vi "PrepareXYSignals.vi"(8 "error in (no error)":errorcluster, 9 "Parameters":T2={"number of planes"=4, "z step"=1.9999999999999998e-05, "pixel dwell time"=1.0000000000000001e-11, "z frequency"=10.0, "number of pixels"=100, "smooth points"=10, "smooth line"=10, "Sine\nSawtooth"=FALSE, "PointSorting"=0, "Sort Points"=FALSE, "X-pixels"=256.0, "Y-lines"=256.0, "pixelstoµm"=256.0, "zoom"=1.0, "Time offset"=1.0000000000000001e-11} {"zoom" min=0.5 step=0.1; "Y-lines" min=1 step=1; "X-pixels" min=1 step=1; "PointSorting" items=["No Difference", "Every Second Point", "Down / Up"]; "smooth line" min=1; "smooth points" min=1; "number of pixels" min=1; "z frequency" format="%_4g"; "number of planes" min=1}, 10 "DutyCluster":T1 {"Iteration" items=["first iteration", "second iteration"]}, 11 "XYZ Point coordinates (pixels)":dbl[][](array[numeric])) -> (0 "error out":errorcluster, 2 "DutyCluster":T1 {"Iteration" items=["first iteration", "second iteration"]}, 3 "XY Point coordinates (um)":dbl[][](array[numeric]))   [LabVIEW 2010]
uses:
  TypeDefs/DutyCluster.ctl
  TypeDefs/ParameterCluster.ctl
  <vilib>/Analysis/_algsub.llb/Real Vector Norm.vi
  <vilib>/Analysis/NI_AALPro.lvlib
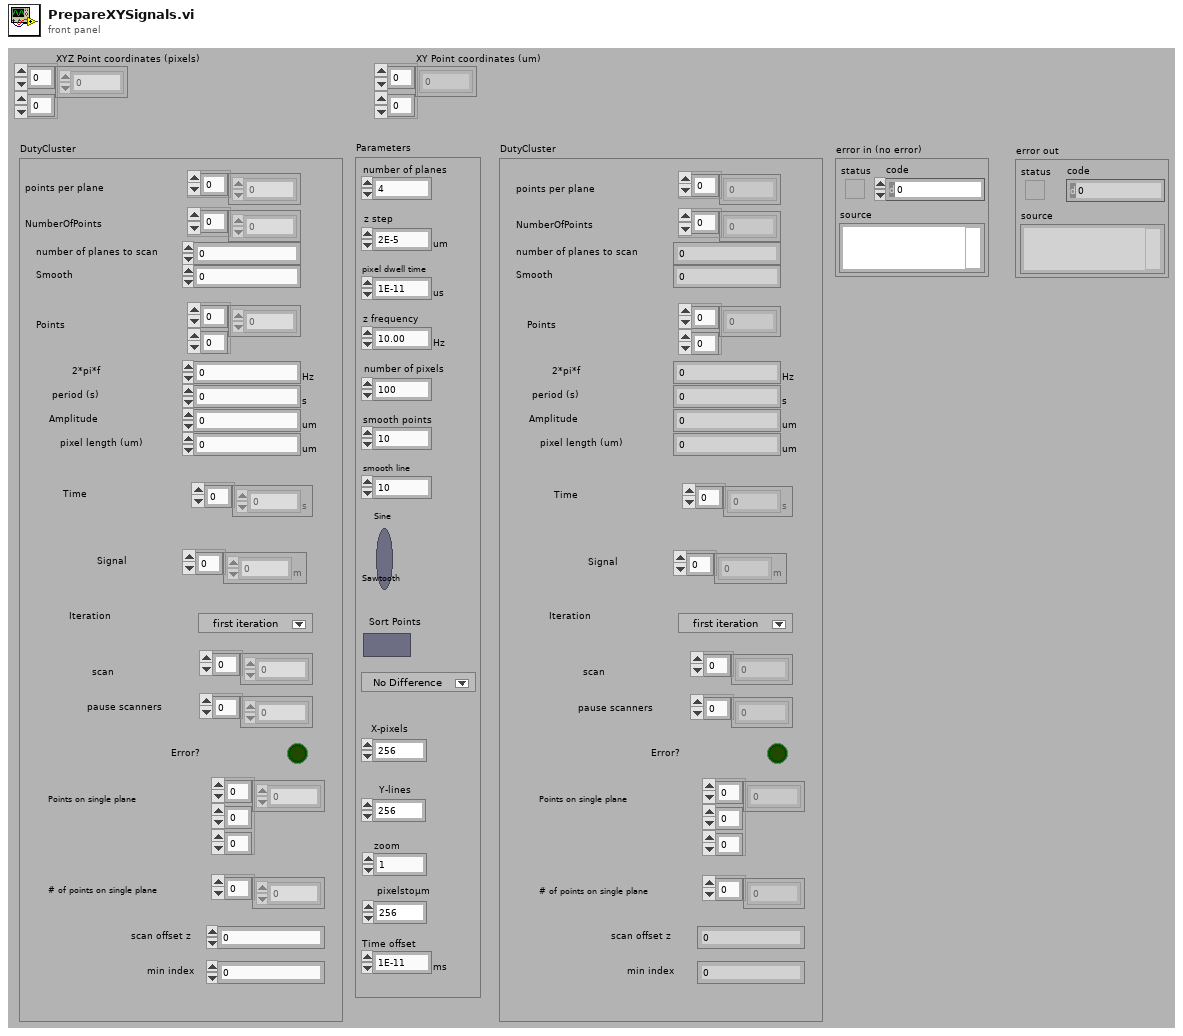
[diagram p1: front panel]
types:
  T1 = typedef "DutyCluster.ctl" = cluster{"points per plane":i32[], "NumberOfPoints":i32[], "number of planes to scan":i32, "Smooth":i32, "Points":dbl[][], "2*pi*f":dbl[unit], "period (s)":dbl[unit], "Amplitude":dbl[unit], "pixel length (um)":dbl[unit], "Time":dbl[unit][], "Signal":dbl[unit][], "Iteration":u16, "scan":i32[], "pause scanners":i32[], "Error?":bool, "Points on single plane":dbl[][][], "# of points on single plane":i32[], "scan offset z":i32, "min index":i32}
  T2 = typedef "ParameterCluster.ctl" = cluster{"number of planes":i32, "z step":dbl[unit], "pixel dwell time":dbl[unit], "z frequency":dbl[unit], "number of pixels":i32, "smooth points":i32, "smooth line":i32, "Sine\nSawtooth":bool, "PointSorting":u16, "Sort Points":bool, "X-pixels":sgl, "Y-lines":sgl, "pixelstoµm":dbl, "zoom":dbl, "Time offset":dbl[unit]}
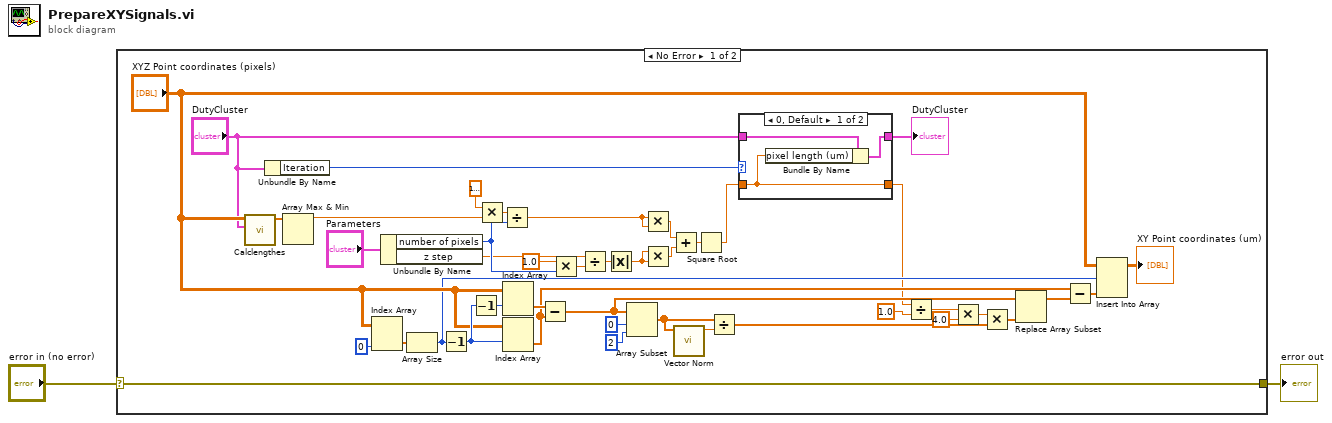
[diagram p0: block diagram]
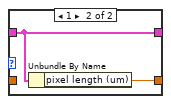
[diagram p2: hidden frame]
diagram:
  n1 = case shown="No Error" "error in (no error)" {
    selector: "error in (no error)" -> [w6 w51]
    tunnel: [w6 w51] -> w1
    frame No Error {
      n2 = call "Calclengthes.vi"("DutyCluster"="DutyCluster", "XYZ coordinates (um)"="XYZ Point coordinates (pixels)") -> ("difference"=w45:dbl[])  [unwired: 6 in, 1 out]
      n3 = Unbundle By Name("DutyCluster") -> ("Iteration"=w12:u16)
      n4 = Array Max & Min(array=w45) -> (max value=w41:dbl)  [unwired: 3 out]
      n5 = Index Array(array="XYZ Point coordinates (pixels)", index (col)=0 ("disabled index (col)")) -> (element=w35:dbl[])  [unwired: 1 in]
      n6 = Unbundle By Name("Parameters") -> ("number of pixels"=w26:i32, "z step"=w25:dbl[unit])
      n7 = Array Size(array=w35) -> (size(s)=w13:i32)
      n8 = Decrement(x=w13) -> (x-1=w34:i32)
      n9 = Decrement(x=w34) -> (x-1=w33:i32)
      n10 = Multiply(x=dbl[unit] 1e-06, y=w41) -> (x*y=w40:dbl[unit])
      n11 = Divide(x=w40, y=w26) -> (x/y=w42:dbl[unit])
      n12 = Index Array(array="XYZ Point coordinates (pixels)", index (row)=w33) -> (element=w37:dbl[])  [unwired: 1 in]
      n13 = Index Array(array="XYZ Point coordinates (pixels)", index (row)=w34) -> (element=w16:dbl[])  [unwired: 1 in]
      n14 = Subtract(x=w37, y=w16) -> (x-y=w17:dbl[])
      n15 = Multiply(x=1.0, y=w26) -> (x*y=w30:dbl)
      n16 = Divide(x=w25, y=w30) -> (x/y=w29:dbl[unit])
      n17 = Absolute Value(x=w29) -> (abs(x)=w28:dbl[unit])
      n18 = Array Subset(array=w17, index=0, length=2) -> (w4:dbl[])
      n19 = Multiply(x=w42, y=w42) -> (x*y=w44:dbl[unit])
      n20 = Multiply(x=w28, y=w28) -> (x*y=w43:dbl[unit])
      n21 = Add(x=w44, y=w43) -> (x+y=w15:dbl[unit])
      n22 = call-poly <vilib>:"Vector Norm.vi"("Input Vector"=w4) -> ("norm"=w3:dbl)  [unwired: 9 in, 1 out]
      n23 = Square Root(x=w15) -> (sqrt(x)=w19:dbl[unit])
      n24 = Divide(x=w4, y=w3) -> (x/y=w18:dbl[])
      n25 = case shown="0, Default" w12 {
        tunnel: w19 -> [w48 _]
        tunnel: [w48 w50] -> w8
        tunnel: "DutyCluster" -> [w47 w49]
        tunnel: [w46 w49] -> w5
        frame 0, Default {
          n26 = Bundle By Name(cluster=w47, "pixel length (um)"=w48) -> (w46:T1)
        }
        frame 1 {
          n27 = Unbundle By Name(w49) -> ("pixel length (um)"=w50:dbl[unit])
        }
      }
      "DutyCluster" <- w5
      n28 = Divide(x=w8, y=dbl[unit] 1.0) -> (x/y=w9:dbl)
      n29 = Multiply(x=w9, y=4.0) -> (x*y=w21:dbl)
      n30 = Multiply(x=w21, y=w18) -> (x*y=w20:dbl[])
      n31 = Replace Array Subset(array=w17, new element=w20) -> (w23:dbl[])  [unwired: 1 in]
      n32 = Subtract(x=w16, y=w23) -> (x-y=w24:dbl[])
      n33 = Insert Into Array(array="XYZ Point coordinates (pixels)", index (row)=w13, new element=w24) -> (→"XY Point coordinates (um)":dbl[][])  [unwired: 1 in]
    }
    frame Error {
    }
  }
  "error out" <- w1
